vi "dataAcq_X_wnr_create.vi"(0 "x scale in, (WNr, THz, )":sgl[](array[numeric]) format="%.2f", 1 "x_min":sgl format="%^.3e", 2 "x_max":sgl format="%^.3e", 4 "points":u32, 5 "error in (no error)":errorcluster) -> (14 "x scale out":sgl[](array[numeric]) format="%.2f", 19 "error out":errorcluster)   [LabVIEW 2010, in "OSA.lvclass"]
uses:
  OSA.lvclass
panel:
  out "x/y":ext format="%^.3e"
  out "single precision float":sgl format="%^.3e"
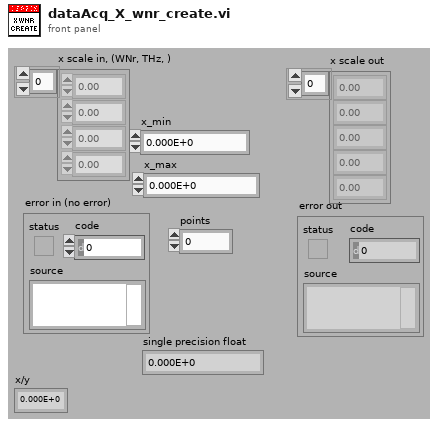
[diagram p1: front panel]
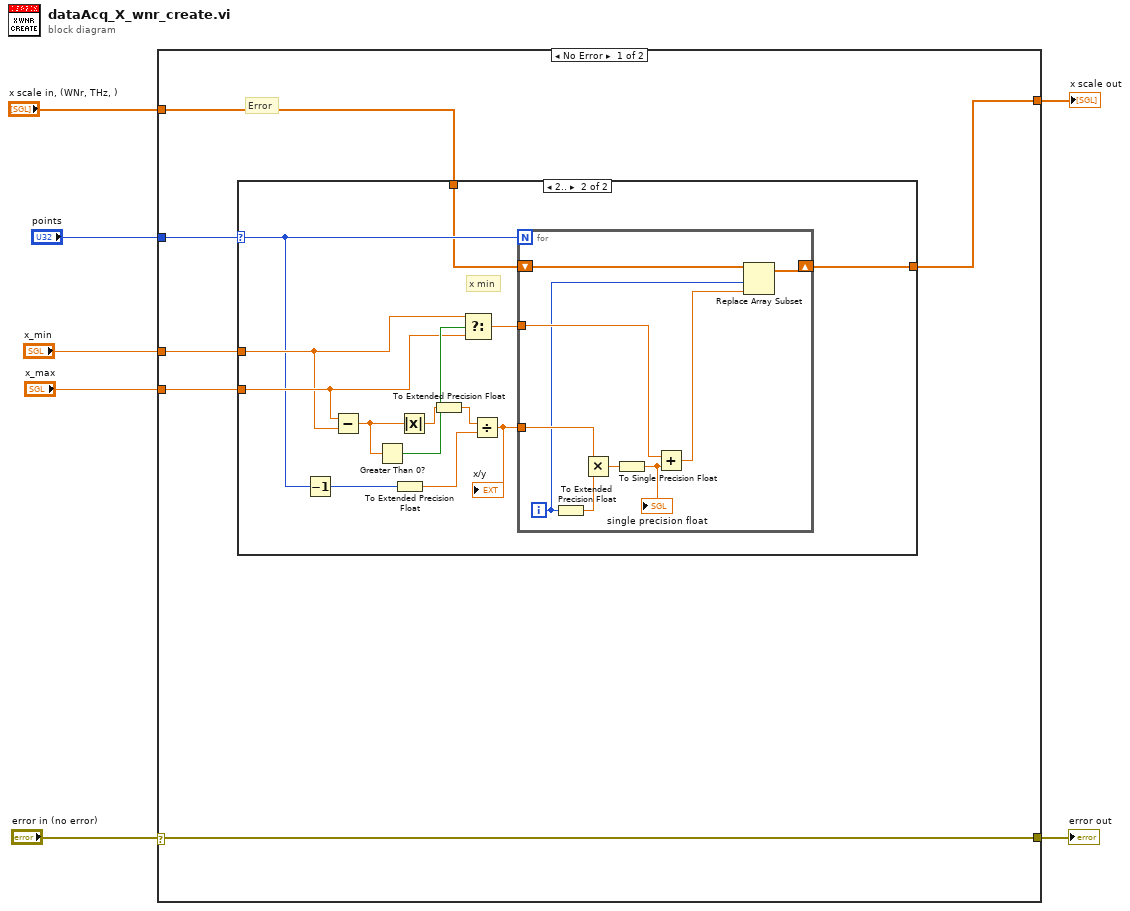
[diagram p0: block diagram]
diagram:
  n1 = case shown="No Error" "error in (no error)" {
    selector: "error in (no error)" -> [w13 w37]
    tunnel: [w13 w37] -> w7
    tunnel: "points" -> [w12 _]
    tunnel: "x_min" -> [w11 _]
    tunnel: "x_max" -> [w10 _]
    tunnel: "x scale in, (WNr, THz, )" -> [w9 w38]
    tunnel: [w8 w38] -> w1
    frame No Error {
      # "Error"
      n2 = case shown="2.." w12 {
        selector: w12 -> [_ w22]
        tunnel: w11 -> [_ w24]
        tunnel: w10 -> [_ w25]
        tunnel: w9 -> [w14 w17]
        tunnel: [w14 w16] -> w8
        frame 0, Default {
        }
        frame 2.. {
          # "x min"
          n3 = Decrement(x=w22) -> (x-1=w15:u32)
          n4 = Subtract(x=w25, y=w24) -> (x-y=w27:sgl)
          n5 = Greater Than 0?(x=w27) -> (x > 0?=w26:bool)
          n6 = To Extended Precision Float(1:w15) -> (0:w18:ext)
          n7 = Absolute Value(x=w27) -> (abs(x)=w20:sgl)
          n8 = To Extended Precision Float(1:w20) -> (0:w19:ext)
          n9 = Select(t=w24, s=w26, f=w25) -> (s? t:f=w23:sgl)
          n10 = Divide(x=w19, y=w18) -> (x/y=w21:ext)
          "x/y" <- w21
          n11 = for {
            N: w22 -> [_]
            tunnel: w23 -> [w32]
            tunnel: w21 -> [w36]
            shift-right: [w30] -> w16
            shift-left: w17 -> [w31]
            i -> [w29]
            n12 = To Extended Precision Float(1:w29) -> (0:w33:ext)
            n13 = Multiply(x=w36, y=w33) -> (x*y=w35:ext)
            n14 = To Single Precision Float(number=w35) -> (single precision float=w34:sgl)
            "single precision float" <- w34
            n15 = Add(x=w32, y=w34) -> (x+y=w28:sgl)
            n16 = Replace Array Subset(array=w31, new element=w28, index=w29) -> (w30:sgl[])
          }
        }
      }
    }
    frame Error {
      # "Put your own code here"
    }
  }
  "error out" <- w7
  "x scale out" <- w1
